vi "RoomStateToUI.vi"(8 "error in":errorcluster, 11 "Room In":refnum<class "Room.lvclass">) -> (0 "error out":errorcluster, 2 "Selected Room":T1={"Room Number"=0, "RoomNumFlags"={"Flag State"=[1, 3, 5, 7]}, "BedVacant"=FALSE, "InRoomPersonnel"=[], "RoomRequests"=[]}, 3 "Room Out":refnum<class "Room.lvclass">)   [LabVIEW 2015, in "Room.lvclass"]
uses:
  Room.lvclass
  NurseStation/TypeDef/SelectedRoom.ctl
  Flags/ColorFlags.ctl
  Room.lvclass/Room.ctl
  Read Flags.lvclass.vi
  Read BedVacant.vi
  Read InRoomPersonnel.vi
  Read RoomRequests.vi
  Read Room Number.vi
  Flags/Flags.lvclass
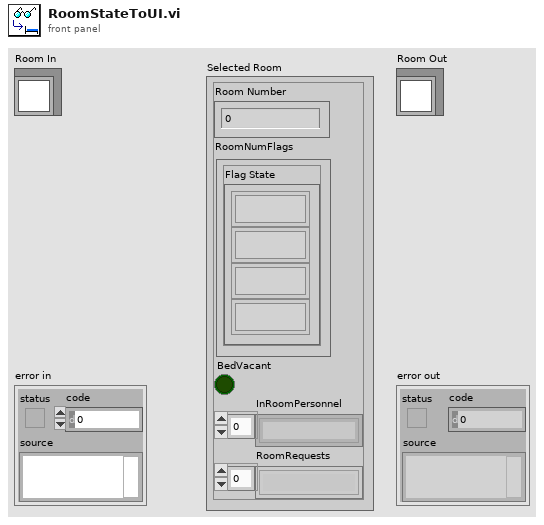
[diagram p1: front panel]
types:
  T1 = typedef "Room.lvclass/SelectedRoom.ctl" = cluster{"Room Number":u8, "RoomNumFlags":T2, "BedVacant":bool, "InRoomPersonnel":string[], "RoomRequests":string[]}
  T2 = typedef "Flags.lvclass/ColorFlags.ctl" = cluster{"Flag State":u8[]}
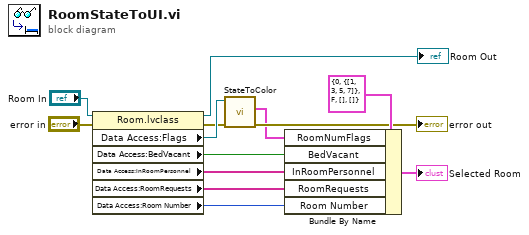
[diagram p0: block diagram]
diagram:
  n1 = property class="Room.lvclass"(reference="Room In", error in="error in") -> (reference out=→"Room Out":refnum<class "Room.lvclass">, error out=w10:errorcluster, "Data Access:Flags"=w11:refnum<class "Flags.lvclass">, "Data Access:BedVacant"=w7:bool, "Data Access:InRoomPersonnel"=w1:string[], "Data Access:RoomRequests"=w2:string[], "Data Access:Room Number"=w3:i32)
  n2 = call "StateToColor.vi"("error in (no error)"=w10, "Flags in"=w11) -> ("error out"=→"error out":errorcluster, "RoomNumFlags"=w6:T2)  [unwired: 7 in, 1 out]
  n3 = Bundle By Name(cluster=T1 {"Room Number"=0, "RoomNumFlags"={"Flag State"=[1, 3, 5, 7]}, "BedVacant"=FALSE, "InRoomPersonnel"=[], "RoomRequests"=[]} ("Selected Room"), "RoomNumFlags"=w6, "BedVacant"=w7, "InRoomPersonnel"=w1, "RoomRequests"=w2, "Room Number"=w3) -> (→"Selected Room":T1)
